vi "SRV_VIG_Movie.vi"(9 "Images Directory Path":path, 12 "Method (Get)":enum16{"Get", "Start", "Stop"}(ring)) -> (4 "Movie?":bool, 6 "Timestamp String out":string, 8 "Count out":i32, 10 "Images Directory Path out":path)   [LabVIEW 2014]
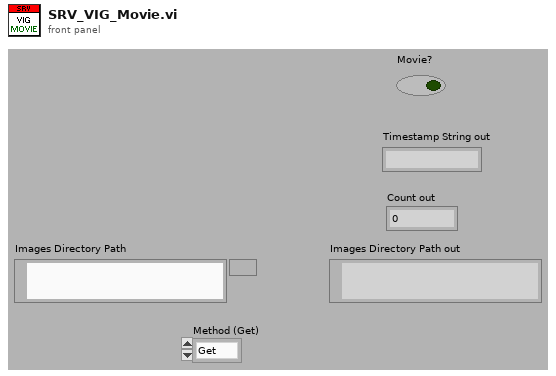
[diagram p1: front panel]
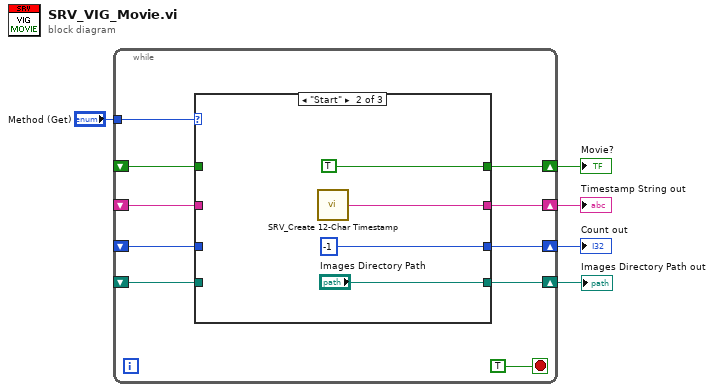
[diagram p0: block diagram]
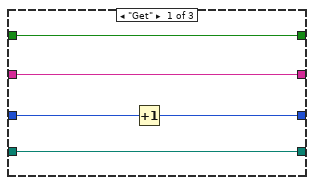
[diagram p2: hidden frame]
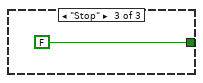
[diagram p3: hidden frame]
diagram:
  n1 = while {
    tunnel: "Method (Get)" -> [w15]
    shift-right: [w13] -> w4
    shift-left: _ -> [w14]
    shift-right: [w11] -> w3
    shift-left: _ -> [w10]
    shift-right: [w9] -> w2
    shift-left: _ -> [w8]
    shift-right: [w7] -> w1
    shift-left: _ -> [w6]
    stop <- TRUE stop-if-true
    n2 = case shown="\"Start\"" w15 {
      tunnel: w14 -> [w20 _ _]
      tunnel: [w20 TRUE ("Movie?") FALSE ("Movie?")] -> w13
      tunnel: [w19 w24 _] -> w11
      tunnel: w10 -> [w19 _ _]
      tunnel: [w17 -1 ("Count") _] -> w9
      tunnel: w8 -> [w18 _ _]
      tunnel: [w16 "Images Directory Path" _] -> w7
      tunnel: w6 -> [w16 _ _]
      frame "Get" {
        n3 = Increment(x=w18) -> (x+1=w17:i32)
      }
      frame "Start" {
        n4 = call "SRV_Create 12-Char Timestamp.vi"() -> ("Timestamp String"=w24:string)  [unwired: 15 in]
      }
      frame "Stop" {
      }
    }
  }
  "Movie?" <- w4
  "Timestamp String out" <- w3
  "Count out" <- w2
  "Images Directory Path out" <- w1
